vi "Temperature Logger V2.vi"() -> ()   [LabVIEW 2021]
uses:
  <vilib>/Analysis/Matrix/Datatypes/RealMatrix.ctl
  <vilib>/Utility/file.llb/Read Delimited Spreadsheet (DBL).vi
  <vilib>/Analysis/Matrix/Numeric/Conversions/Matrix To Array - RM.vi
  <vilib>/Utility/file.llb/Write Delimited Spreadsheet (DBL).vi
  <vilib>/gmath/NI_Gmath.lvlib
  <vilib>/Analysis/Matrix/NI_Matrix.lvlib
  <vilib>/Analysis/NI_AALBase.lvlib
panel:
  in  "Tab Control":enum32{"Automatic", "Override"}(tab)
  in  "Enable":bool[](array[boolean])=[TRUE, TRUE, TRUE, FALSE, FALSE, FALSE, FALSE, FALSE]
  in  "Read Time":u16[](array[ring])=[30, 30, 30, 30, 30, 30, 30, 30] items=["2 h"=7200, "1 h"=3600, "30 m"=1800, "20 m"=1200, "10 m"=600, "5 m"=300, "2 m"=120, "1 m"=60, "30 s"=30]
  in  "Excitation":u8[](array[ring])=[4, 4, 4, 4, 4, 4, 4, 4] items=["3 mV"=7, "1 mV"=6, "300 uV"=5, "100 uV"=4, "30 uV"=3, "10 uV"=2, "3 uV"=1, "0"=0]
  in  "Measure Now":bool[](array[boolean])=[FALSE, FALSE, FALSE, FALSE, FALSE, FALSE, FALSE, FALSE]
  out "Last Resistance":dbl[](array[numeric])
  in  "VISA RESOURCE":refnum<visa-resource-name>="COM5"
  in  "Override":bool
  out "Raw Resistance":dbl
  in  "FAA Channel":i32(ring) items=["7"=7, "6"=6, "5"=5, "4"=4, "3"=3, "2"=2, "1"=1, "0"=0]
  in  "GGG Channel":i32(ring)=2 items=["7"=7, "6"=6, "5"=5, "4"=4, "3"=3, "2"=2, "1"=1, "0"=0]
  out "FAA Temp":dbl format="%#_4g"
  out "GGG Temp":dbl format="%#_4g"
  out "GGG Resistance":dbl format="%0.2f"
  out "FAA Resistance":dbl format="%0.2f"
  in  "Moving Median Size":i32=35
  in  "Temperature Log File Path":path
  in  "GGG Calibration File":path
  in  "FAA Calibration FIle":path
  in  "lHe Channel":i32(ring)=1 items=["7"=7, "6"=6, "5"=5, "4"=4, "3"=3, "2"=2, "1"=1, "0"=0]
  out "lHe Temp":dbl format="%#_4g"
  out "lHe Resistance":dbl format="%0.2f"
  in  "lHe Calibration File":path
  out "Currenty Measuring":dbl(knob) max=1.0 scale=0.0..2.0
  in  "Override Controls":T1
  out "Temperature Plot":cluster{timestamp[], dbl[]}[](graph)
  # "Channel 0:"
  # "Channel 1:"
  # "Channel 2:"
  # "Channel 3:"
  # "Channel 4:"
  # "Channel 5:"
  # "Channel 6:"
  # "Channel 7:"
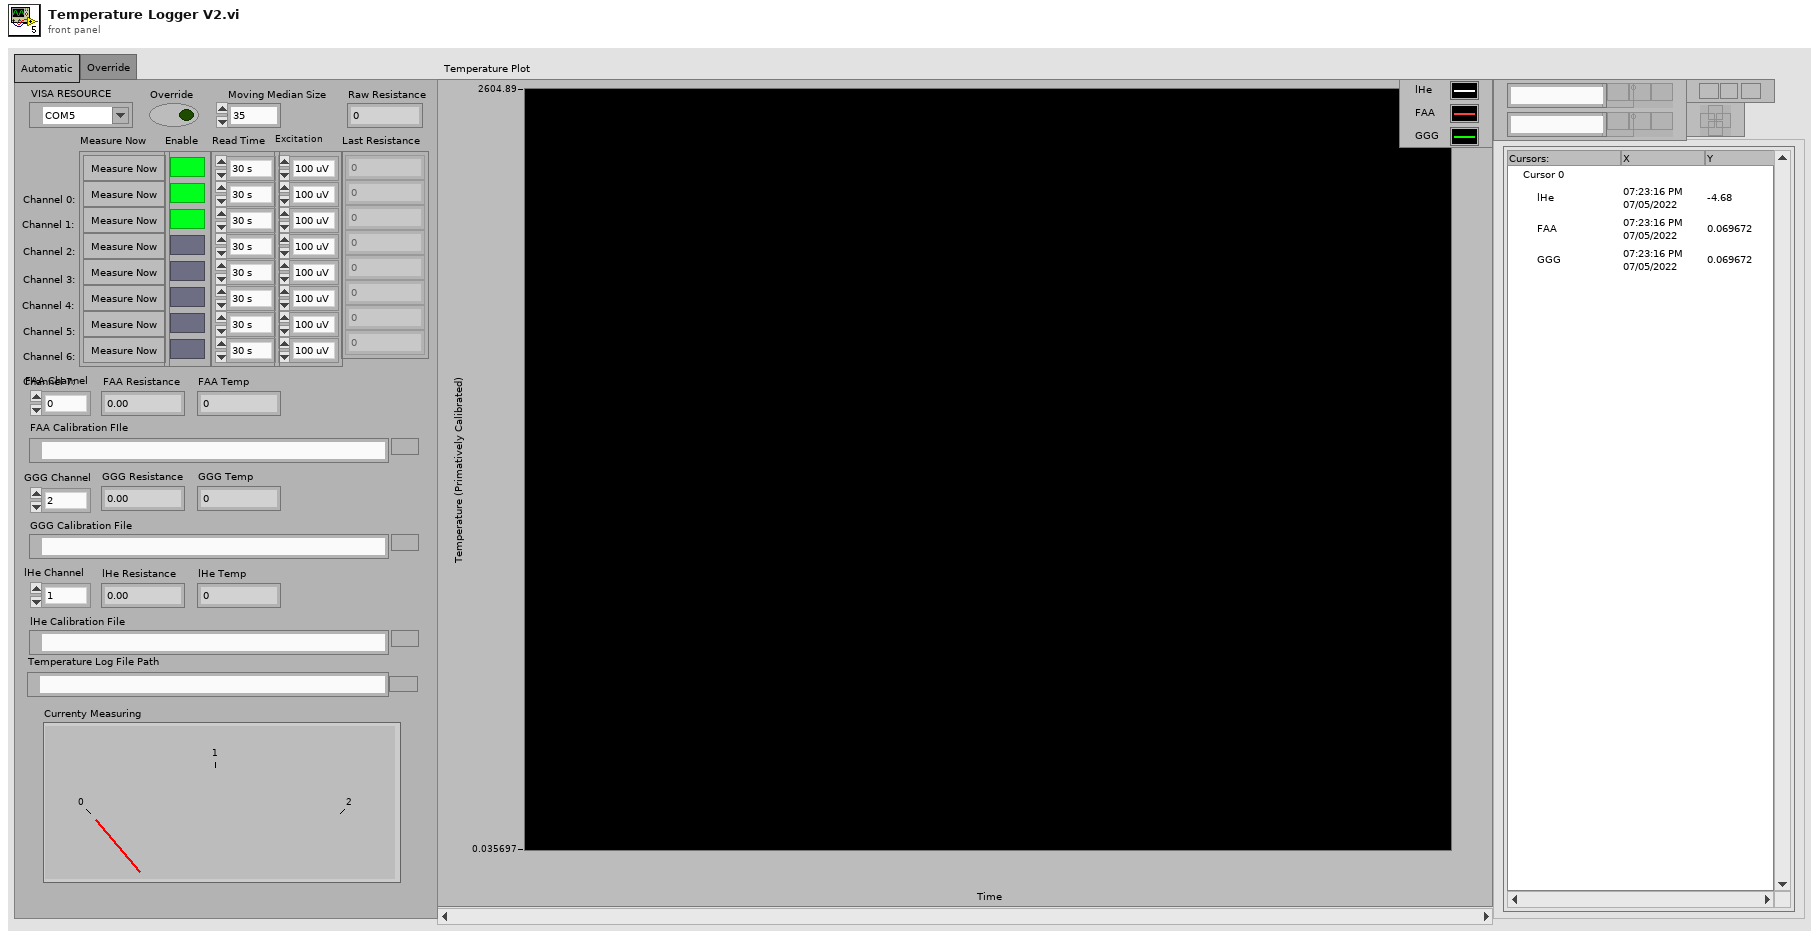
[diagram p1: front panel]
types:
  T1 = cluster{"VISA RESOURCE":refnum<visa-resource-name>, "PICOBUS ADDRESS":u8, "DISABLE AL":u8, "REMOTE":u8, "INPUT":u8, "CHANNEL":u8, "RANGE":u8, "EXCITATION":u8, "DISPLAY":u8, "DIGITAL\nREFERENCE":u16, "SET POINT":dbl, "PROP GAIN":u8, "INTG":u8, "DERIV":u8, "POWER BIAS":u8, "POWER RANGE":u8, "INFO STRING":string, "HEATER\nRESISTANCE":dbl, "INTERVAL":u8, " SENSOR dR/dT":u8}
  T2 = typedef "NI_Matrix.lvlib/RealMatrix.ctl" = dbl[][]
  T3 = cluster{"VISA RESOURCE":refnum<visa-resource-name>, "PICOBUS ADDRESS":u8, "DISABLE AL":u8, "REMOTE":u8, "INPUT":u8, "CHANNEL":u8, "RANGE":u8, "EXCITATION":u8, "DISPLAY":u8, "DIGITAL REFERENCE":u16, "SET POINT":dbl, "PROP GAIN":u8, "INTG":u8, "DERIV":u8, "POWER BIAS":u8, "POWER RANGE":u8, "INFO STRING":string, "HEATER RESISTANCE":dbl, "INTERVAL":u8, " SENSOR dR/dT":u8}
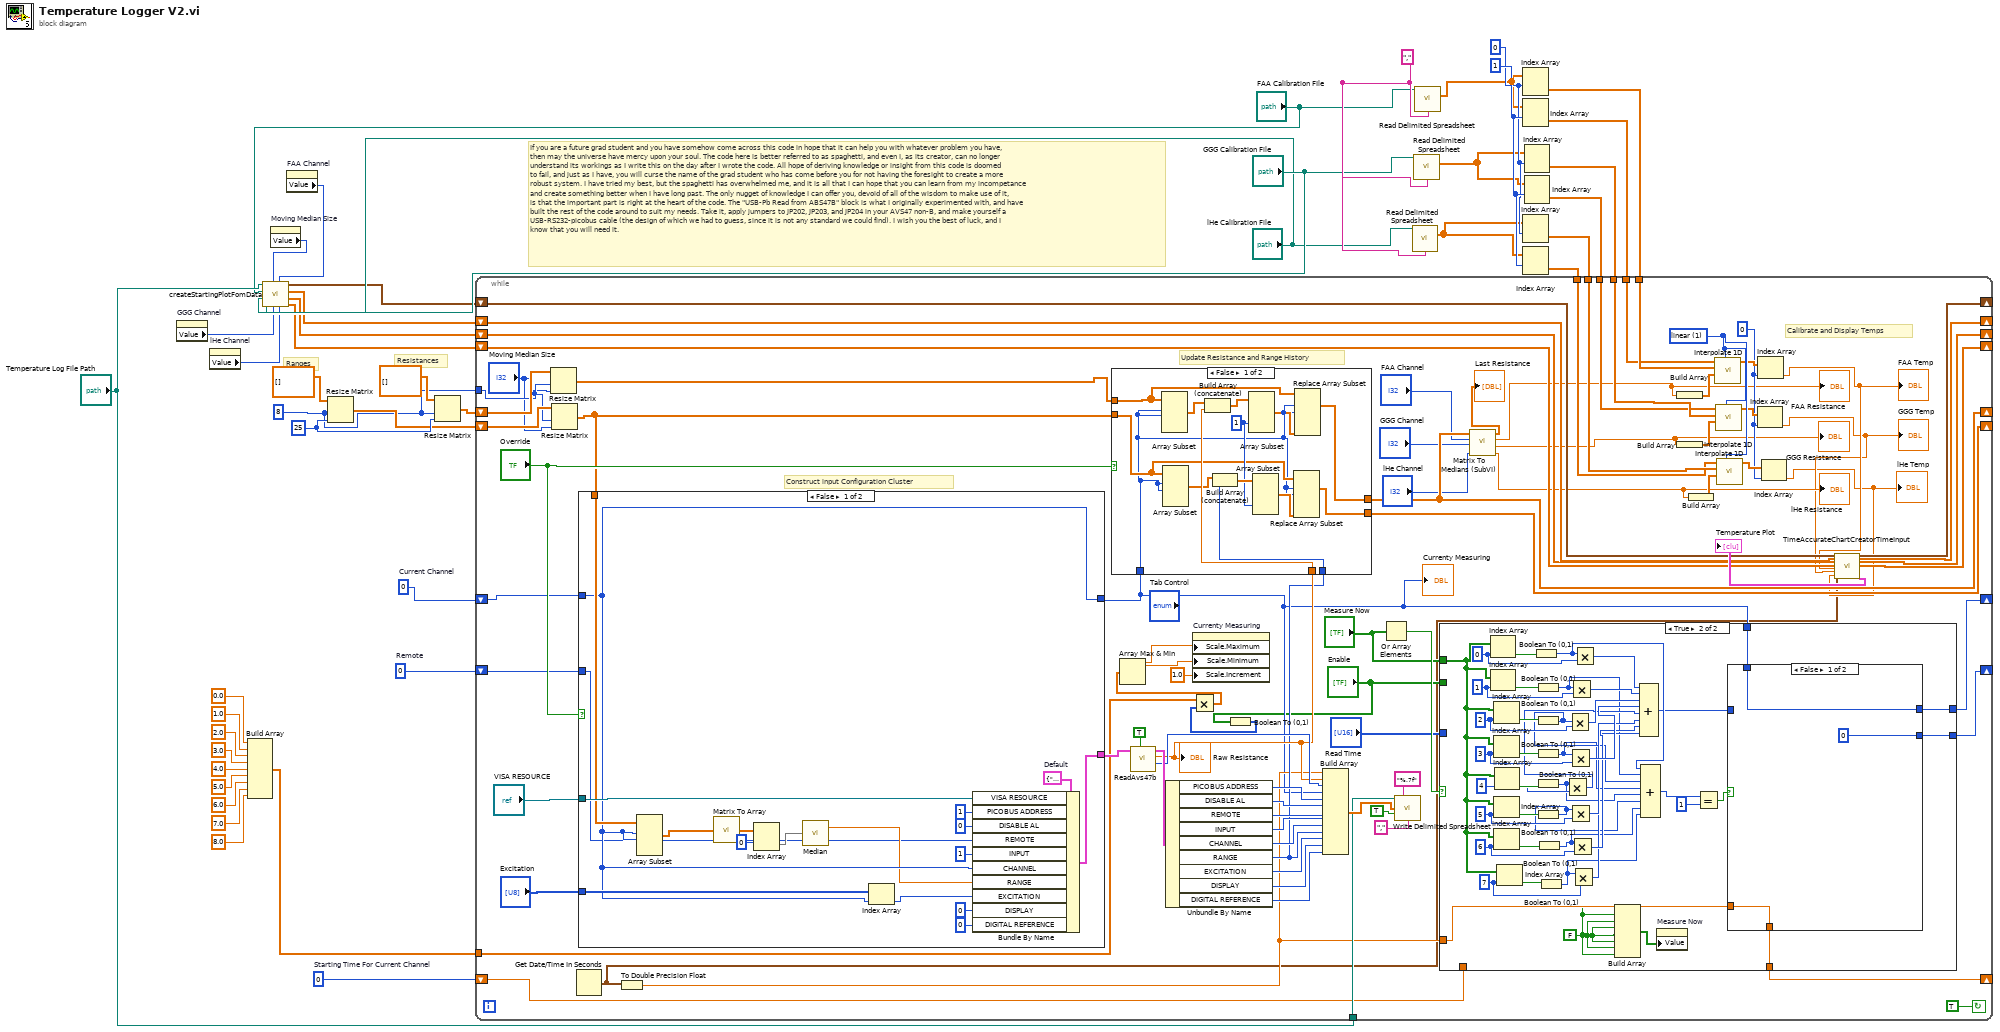
[diagram p0: block diagram]
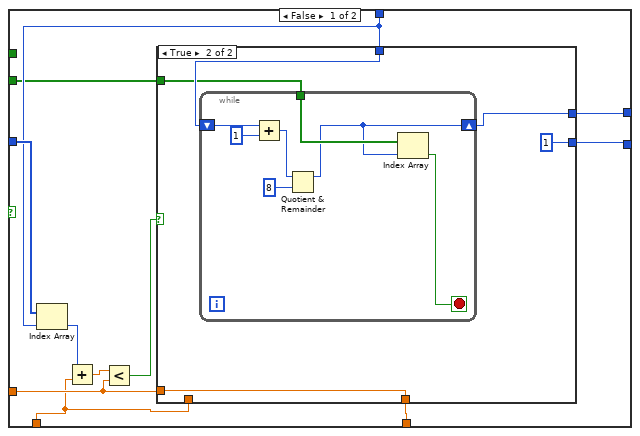
[diagram p2: hidden frame]
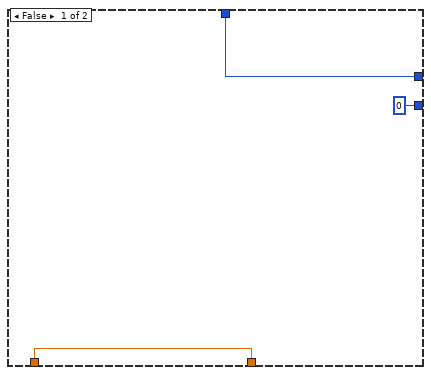
[diagram p3: hidden frame]
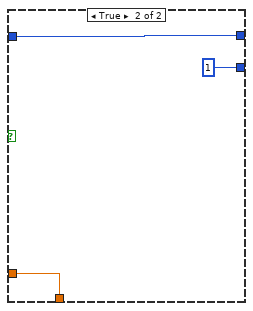
[diagram p4: hidden frame]
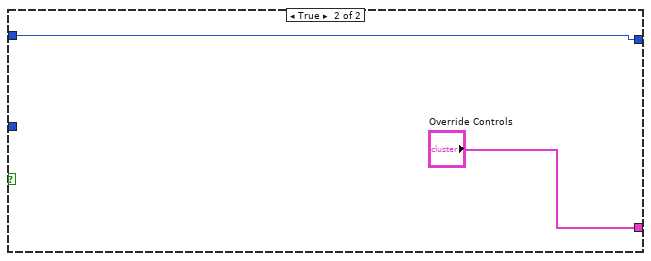
[diagram p5: hidden frame]
diagram:
  w24 = 0  # Remote
  w27 = 25 ("number of columns")
  w25 = 8 ("number of rows")
  w23 = 0  # Starting Time For Current Channel
  w31 = 0  # Current Channel
  w42 = 1 ("index (row)")
  w41 = 0 ("index (row)")
  w43 = "," ("delimiter (\\t)")
  # "If you are a future grad student and you have somehow come across this code in hope that it can help you with whatever problem you have,\nthen may the universe have mercy upon your soul. The code here is better referred to as spaghetti, and even I, as its creator, can no longer\nunderstand its workings as I write this on the day after I wrote the code. All hope of deriving knowledge or insight from this code is doomed\nto fail, and just as I have, you will curse the name of the grad student who has come before you for not having the foresight to create a more\nrobust system. I have tried my best, but the spaghetti has overwhelmed me, and it is all that I can hope that you can learn from my incompetance\nand create something better when I have long past. The only nugget of knowledge I can offer you, devoid of all of the wisdom to make use of it,\nis that the important part is right at the heart of the code. The \"USB-Pb Read from ABS47B\" block is what I originally experimented with, and have\nbuilt the rest of the code around to suit my needs. Take it, apply jumpers to JP202, JP203, and JP204 in your AVS47 non-B, and make yourself a\nUSB-RS232-picobus cable (the design of which we had to guess, since it is not any standard we could find). I wish you the best of luck, and I\nknow that you will need it."
  # "Ranges"
  # "Resistances"
  n1 = property on="GGG Channel" class="Ring (strict)"() -> ("Value"=w2:i32)  [unwired: 2 in, 2 out]
  n2 = property on="lHe Channel" class="Ring (strict)"() -> ("Value"=w1:i32)  [unwired: 2 in, 2 out]
  n3 = Build Array(0.0 ("element"), 1.0 ("element"), 2.0 ("element"), 3.0 ("element"), 4.0 ("element"), 5.0 ("element"), 6.0 ("element"), 7.0 ("element"), 8.0 ("element")) -> (w13:dbl[])
  n4 = property on="Moving Median Size" class="DigNum (strict)"() -> ("Value"=w4:i32)  [unwired: 2 in, 2 out]
  n5 = property on="FAA Channel" class="Ring (strict)"() -> ("Value"=w3:i32)  [unwired: 2 in, 2 out]
  n6 = call "createStartingPlotFomData.vi"("lHe Channel"=w1, "FAA Channel"=w3, "GGG Channel"=w2, "Moving Median Size"=w4, "lHe Calibration File"="lHe Calibration File", "GGG Calibration File"="GGG Calibration File", "FAA Calibration FIle"="FAA Calibration FIle", "Temperature Log File Path 2"="Temperature Log File Path") -> ("4K Plot Data"=w5:dbl[], "GGG Plot Data"=w6:dbl[], "FAA Plot Data"=w7:dbl[], "Time Plot Data"=w8:timestamp[])
  n7 = Resize Matrix(1:w27, 2:w25, 4:T2 [] ("matrix")) -> (0:w26:T2)
  n8 = Resize Matrix(1:w27, 2:w25, 4:T2 [] ("matrix")) -> (0:w28:T2)
  n9 = call-poly <vilib>:"Read Delimited Spreadsheet.vi"("file path (dialog if empty)"="lHe Calibration File", "delimiter (\\t)"=w43) -> ("all rows"=w38:dbl[][])  [unwired: 8 in, 5 out]
  n10 = call-poly <vilib>:"Read Delimited Spreadsheet.vi"("file path (dialog if empty)"="GGG Calibration File", "delimiter (\\t)"=w43) -> ("all rows"=w39:dbl[][])  [unwired: 8 in, 5 out]
  n11 = call-poly <vilib>:"Read Delimited Spreadsheet.vi"("file path (dialog if empty)"="FAA Calibration FIle", "delimiter (\\t)"=w43) -> ("all rows"=w40:dbl[][])  [unwired: 8 in, 5 out]
  n12 = Index Array(array=w40, index (row)=w41) -> (element=w37:dbl[])  [unwired: 1 in]
  n13 = Index Array(array=w40, index (row)=w42) -> (element=w36:dbl[])  [unwired: 1 in]
  n14 = Index Array(array=w38, index (row)=w41) -> (element=w33:dbl[])  [unwired: 1 in]
  n15 = Index Array(array=w38, index (row)=w42) -> (element=w32:dbl[])  [unwired: 1 in]
  n16 = Index Array(array=w39, index (row)=w41) -> (element=w35:dbl[])  [unwired: 1 in]
  n17 = Index Array(array=w39, index (row)=w42) -> (element=w34:dbl[])  [unwired: 1 in]
  n18 = while {
    tunnel: w37 -> [w116]
    tunnel: w36 -> [w115]
    tunnel: w35 -> [w114]
    tunnel: w34 -> [w113]
    tunnel: w33 -> [w112]
    tunnel: w32 -> [w111]
    shift-right: [w106] -> _
    shift-left: w8 -> [w110]
    shift-right: [w104] -> _
    shift-left: w5 -> [w107]
    shift-right: [w105] -> _
    shift-left: w7 -> [w109]
    shift-right: [w71] -> _
    shift-left: w6 -> [w108]
    shift-right: [w61] -> _
    shift-left: w31 -> [w68]
    tunnel: "Temperature Log File Path" -> [w88]
    shift-right: [w79] -> _
    shift-left: w28 -> [w87]
    shift-right: [w80] -> _
    shift-left: w26 -> [w86]
    tunnel: w25 -> [w85]
    shift-right: [w60] -> _
    shift-left: w24 -> [w64]
    shift-right: [w56] -> _
    shift-left: w23 -> [w59]
    tunnel: w13 -> [w51]
    stop <- TRUE continue-if-true
    w117 = 0 ("index")
    w123 = 1 items=["nearest", "linear", "spline", "cubic Hermite", "Lagrange"] ("method")
    # "Calibrate and Display Temps"
    # "Update Resistance and Range History"
    # "Construct input Configuration Cluster"
    n19 = Resize Matrix(1:"Moving Median Size", 2:w85, 4:w87) -> (0:w81:T2)
    n20 = Resize Matrix(1:"Moving Median Size", 2:w85, 4:w86) -> (0:w65:T2)
    n21 = Get Date/Time In Seconds() -> (seconds since 1Jan1904=w44:timestamp)
    n22 = case shown="False" "Override" {
      tunnel: [w211 "Override Controls"] -> w69
      tunnel: w68 -> [w209 w221]
      tunnel: [w209 w221] -> w52
      tunnel: "Excitation" -> [w217 _]
      tunnel: "VISA RESOURCE" -> [w212 _]
      tunnel: w65 -> [w210 _]
      tunnel: w64 -> [w204 _]
      frame False {
        w220 = T3 {"VISA RESOURCE"="COM5", "PICOBUS ADDRESS"=1, "DISABLE AL"=0, "REMOTE"=1, "INPUT"=1, "CHANNEL"=0, "RANGE"=5, "EXCITATION"=4, "DISPLAY"=0, "DIGITAL REFERENCE"=0, "SET POINT"=0.0, "PROP GAIN"=0, "INTG"=0, "DERIV"=0, "POWER BIAS"=0, "POWER RANGE"=0, "INFO STRING"="", "HEATER RESISTANCE"=0.0, "INTERVAL"=0, " SENSOR dR/dT"=0}  # Default
        n23 = Array Subset(array=w210, index (row)=w209, length (row)=w209) -> (w203:T2)  [unwired: 2 in]
        n24 = call-poly <vilib>:"Matrix To Array.vi"("Real Matrix"=w203) -> ("Real 2D Array"=w208:dbl[][])
        n25 = Index Array(array=w208, index (row)=0) -> (element=w207:dbl[])  [unwired: 1 in]
        n26 = call <vilib>:"Median.vi"("X"=w207) -> ("median"=w205:dbl)  [unwired: 1 out]
        n27 = Index Array(array=w217, index=w209) -> (element=w216:u8)
        n28 = Bundle By Name(cluster=w220, "VISA RESOURCE"=w212, "PICOBUS ADDRESS"=u8 1, "DISABLE AL"=u8 0, "REMOTE"=w204, "INPUT"=u8 1, "CHANNEL"=w209, "RANGE"=w205, "EXCITATION"=w216, "DISPLAY"=u8 0, "DIGITAL REFERENCE"=u16 0) -> (w211:T3)
      }
      frame True {
      }
    }
    "Currenty Measuring" <- w52
    n29 = To Double Precision Float(number=w44) -> (double precision float=w57:dbl)
    n30 = call "ReadAvs47b.vi"("SYNCHRONISE TO ADC"=TRUE, "CONFIGURATION CLUSTER"=w69) -> ("ADC"=w101:i32, "RESISTANCE (OHMS)"=w83:sgl, "MODIFIED CONFIGURATION CLUSTER"=w102:T3)  [unwired: 4 in, 3 out]
    "Raw Resistance" <- w83
    n31 = Unbundle By Name(w102) -> ("PICOBUS ADDRESS"=w100:u8, "DISABLE AL"=w99:u8, "REMOTE"=w98:u8, "INPUT"=w97:u8, "CHANNEL"=w96:u8, "RANGE"=w82:u8, "EXCITATION"=w95:u8, "DISPLAY"=w94:u8, "DIGITAL REFERENCE"=w93:u16)
    n32 = case shown="False" "Override" {
      tunnel: w83 -> [w235 _]
      tunnel: w82 -> [w233 _]
      tunnel: w81 -> [w229 w238]
      tunnel: w65 -> [w228 w237]
      tunnel: [w224 w238] -> w79
      tunnel: [w225 w237] -> w80
      tunnel: w52 -> [w223 _]
      frame False {
        w230 = 1 ("column 1")
        n33 = Array Subset(array=w229, index (row)=w223, length (row)=w223) -> (w236:T2)  [unwired: 2 in]
        n34 = Array Subset(array=w228, index (row)=w223, length (row)=w223) -> (w234:T2)  [unwired: 2 in]
        n35 = Build Array (concatenate)(w236, w235) -> (w231:T2)
        n36 = Build Array (concatenate)(w234, w233) -> (w232:T2)
        n37 = Array Subset(array=w231, index (col)=w230) -> (w227:T2)  [unwired: 3 in]
        n38 = Array Subset(array=w232, index (col)=w230) -> (w226:T2)  [unwired: 3 in]
        n39 = Replace Array Subset(array=w228, new element=w226, index (dim 0)=w223, index (dim 1)=w223) -> (w225:T2)  [unwired: 2 in]
        n40 = Replace Array Subset(array=w229, new element=w227, index (dim 0)=w223, index (dim 1)=w223) -> (w224:T2)  [unwired: 2 in]
      }
      frame True {
      }
    }
    n41 = Boolean To (0,1)(Boolean="Enable") -> (0, 1=w49:i16[])
    n42 = Multiply(x=w51, y=w49) -> (x*y=w48:dbl[])
    n43 = Array Max & Min(array=w48) -> (max value=w46:dbl, min value=w45:dbl)  [unwired: 2 out]
    n44 = property on="Currenty Measuring" class="Knob (strict)"("Scale.Maximum"=w46, "Scale.Minimum"=w45, "Scale.Increment"=1.0 ("Scale.Range:Minor Increment")) -> ()  [unwired: 2 in, 2 out]
    n45 = Build Array(w57, w83, w101, w52, w100, w99, w98, w97, w96, w82, w95, w94, w93) -> (w89:dbl[])
    n46 = Or Array Elements(Boolean array="Measure Now") -> (logical OR=w63:bool)
    n47 = call-poly <vilib>:"Write Delimited Spreadsheet.vi"("file path (dialog if empty)"=w88, "format (%.3f)"="%.7f", "1D data"=w89, "append to file? (new file:F)"=TRUE, "delimiter (\\t)"="," ("delimiter (\\t)")) -> ()  [unwired: 9 in, 2 out]
    n48 = case shown="True" w63 {
      tunnel: "Measure Now" -> [_ w196]
      tunnel: [w129 w160] -> w61
      tunnel: w52 -> [w128 w158]
      tunnel: [w130 w157] -> w60
      tunnel: w59 -> [w131 _]
      tunnel: "Read Time" -> [w137 _]
      tunnel: w57 -> [w132 w155]
      tunnel: [w133 w156] -> w56
      tunnel: "Enable" -> [w127 _]
      frame False {
        n49 = Index Array(array=w137, index=w128) -> (element=w136:u16)
        n50 = Add(x=w136, y=w131) -> (x+y=w135:dbl)
        n51 = Less?(x=w135, y=w132) -> (x < y?=w134:bool)
        n52 = case shown="True" w134 {
          tunnel: [w140 w145] -> w133
          tunnel: w132 -> [_ w145]
          tunnel: w131 -> [w140 _]
          tunnel: [0 ("Remote") 1 ("Remote")] -> w130
          tunnel: [w138 w141] -> w129
          tunnel: w128 -> [w138 w143]
          tunnel: w127 -> [_ w142]
          frame False {
          }
          frame True {
            n53 = while {
              shift-right: [w146] -> w141
              shift-left: w143 -> [w149]
              tunnel: w142 -> [w151]
              stop <- w150 stop-if-true
              n54 = Add(x=w149, y=1) -> (x+y=w148:i32)
              n55 = Quotient & Remainder(x=w148, y=8) -> (x-y*floor(x/y)=w146:i32)  [unwired: 1 out]
              n56 = Index Array(array=w151, index=w146) -> (element=w150:bool)
            }
          }
        }
      }
      frame True {
        w153 = FALSE
        w180 = 7 ("index")
        w181 = 6 ("index")
        w182 = 5 ("index")
        w183 = 4 ("index")
        w184 = 3 ("index")
        w185 = 2 ("index")
        w186 = 1 ("index")
        w187 = 0 ("index")
        n57 = Index Array(array=w196, index=w187) -> (element=w195:bool)
        n58 = Index Array(array=w196, index=w186) -> (element=w194:bool)
        n59 = Index Array(array=w196, index=w185) -> (element=w193:bool)
        n60 = Index Array(array=w196, index=w184) -> (element=w192:bool)
        n61 = Index Array(array=w196, index=w182) -> (element=w190:bool)
        n62 = Index Array(array=w196, index=w181) -> (element=w189:bool)
        n63 = Index Array(array=w196, index=w183) -> (element=w191:bool)
        n64 = Index Array(array=w196, index=w180) -> (element=w188:bool)
        n65 = Boolean To (0,1)(Boolean=w195) -> (0, 1=w171:i16)
        n66 = Boolean To (0,1)(Boolean=w194) -> (0, 1=w170:i16)
        n67 = Boolean To (0,1)(Boolean=w193) -> (0, 1=w169:i16)
        n68 = Boolean To (0,1)(Boolean=w192) -> (0, 1=w168:i16)
        n69 = Boolean To (0,1)(Boolean=w191) -> (0, 1=w167:i16)
        n70 = Boolean To (0,1)(Boolean=w190) -> (0, 1=w166:i16)
        n71 = Boolean To (0,1)(Boolean=w189) -> (0, 1=w165:i16)
        n72 = Boolean To (0,1)(Boolean=w188) -> (0, 1=w164:i16)
        n73 = Multiply(x=w167, y=w183) -> (x*y=w175:i32)
        n74 = Multiply(x=w169, y=w185) -> (x*y=w177:i32)
        n75 = Multiply(x=w168, y=w184) -> (x*y=w176:i32)
        n76 = Multiply(x=w166, y=w182) -> (x*y=w174:i32)
        n77 = Multiply(x=w170, y=w186) -> (x*y=w178:i32)
        n78 = Multiply(x=w165, y=w181) -> (x*y=w173:i32)
        n79 = Multiply(x=w164, y=w180) -> (x*y=w172:i32)
        n80 = Multiply(x=w171, y=w187) -> (x*y=w179:i32)
        n81 = Build Array(w153, w153, w153, w153, w153, w153, w153, w153) -> (w154:bool[])
        n82 = Compound Arithmetic op=ADD(w179, w178, w177, w176, w175, w174, w173, w172) -> (w159:i32)
        n83 = Compound Arithmetic op=ADD(w171, w170, w169, w168, w167, w166, w165, w164) -> (w163:i16)
        n84 = property on="Measure Now" class="Arr"("Value"=w154) -> ()  [unwired: 2 in, 2 out]
        n85 = Equal?(x=w163, y=i16 1) -> (x = y?=w161:bool)
        n86 = case shown="False" w161 {
          tunnel: [w199 w202] -> w160
          tunnel: w159 -> [_ w202]
          tunnel: w158 -> [w199 _]
          tunnel: [0 ("Remote") 1 ("Remote")] -> w157
          tunnel: [w197 w200] -> w156
          tunnel: w155 -> [w197 w200]
          frame False {
          }
          frame True {
          }
        }
      }
    }
    n87 = call "Matrix To Medians (SubVI).vi"("lHe Channel"="lHe Channel", "GGG Channel"="GGG Channel", "FAA Channel"="FAA Channel", "input matrix"=w79) -> ("lHe Median"=w72:dbl, "GGG Median"=w73:dbl, "FAA median"=w74:dbl, "Resistance Array"=→"Last Resistance":dbl[])  [unwired: 4 in]
    "GGG Resistance" <- w73
    "FAA Resistance" <- w74
    "lHe Resistance" <- w72
    n88 = Build Array(w74) -> (w124:dbl[])
    n89 = Build Array(w73) -> (w122:dbl[])
    n90 = Build Array(w72) -> (w121:dbl[])
    n91 = call <vilib>:"Interpolate 1D.vi"("method"=w123, "xi"=w124, "X"=w116, "Y"=w115) -> ("yi"=w120:dbl[])  [unwired: 5 in, 2 out]
    n92 = call <vilib>:"Interpolate 1D.vi"("method"=w123, "xi"=w122, "X"=w114, "Y"=w113) -> ("yi"=w119:dbl[])  [unwired: 5 in, 2 out]
    n93 = call <vilib>:"Interpolate 1D.vi"("method"=w123, "xi"=w121, "X"=w112, "Y"=w111) -> ("yi"=w118:dbl[])  [unwired: 5 in, 2 out]
    n94 = Index Array(array=w119, index=w117) -> (element=w54:dbl)
    "GGG Temp" <- w54
    n95 = Index Array(array=w120, index=w117) -> (element=w55:dbl)
    "FAA Temp" <- w55
    n96 = Index Array(array=w118, index=w117) -> (element=w53:dbl)
    "lHe Temp" <- w53
    n97 = call "TimeAccurateChartCreatorTimeInput.vi"("Time Shift Reg"=w110, "FAA Shift Reg"=w109, "GGG Shift REg"=w108, "4K Shift Reg"=w107, "FAA Temp"=w55, "GGG Temp"=w54, "lHe Temp"=w53, "current time"=w44) -> ("TIme Out"=w106:timestamp[], "FAA Out"=w105:dbl[], "GGG out"=w71:dbl[], "4K Out"=w104:dbl[], "Temperature Plot"=→"Temperature Plot":cluster{timestamp[], dbl[]}[])  [unwired: 15 in]
  }
